vi "LvIRKit_SUB_GetIRKitIPbyName.vi"(8 "error in (no error)":errorcluster caption="エラー入力（エラーなし）", 11 "IRKit name":string="IRKitA741") -> (0 "error out":errorcluster caption="エラー出力", 1 "IP":string)   [LabVIEW 2014]
uses:
  <vilib>/regexp/Match Regular Expression.xnode
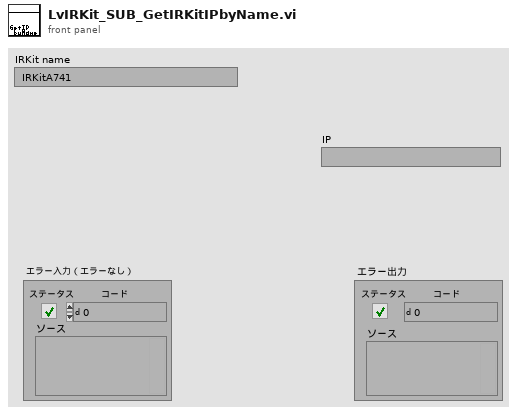
[diagram p1: front panel]
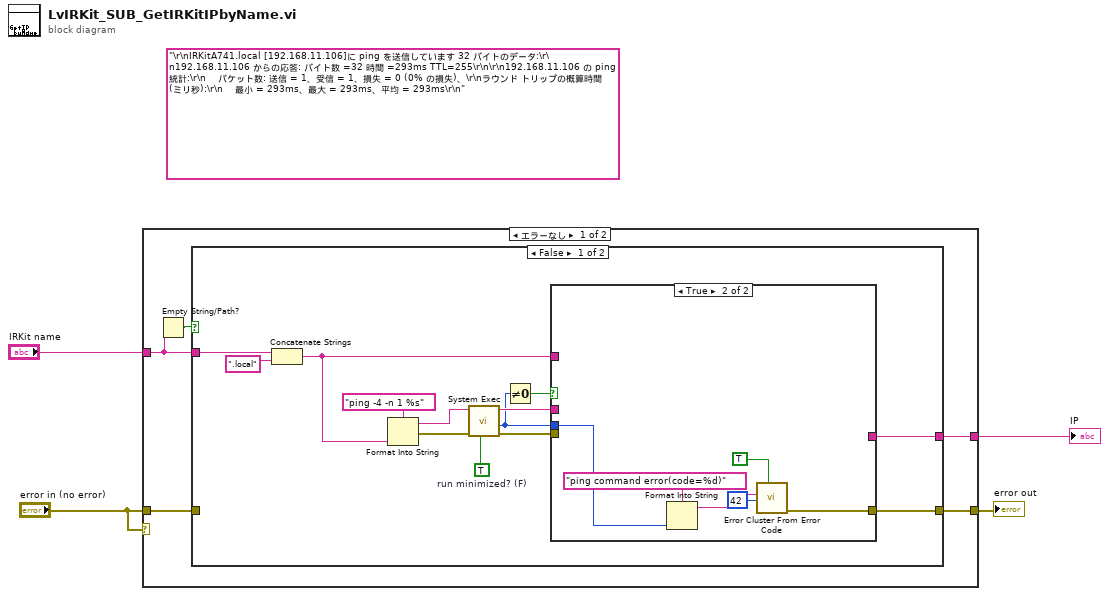
[diagram p0: block diagram]
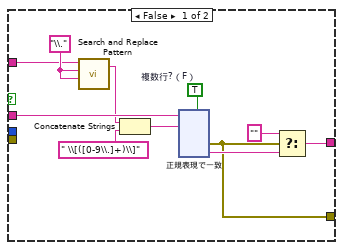
[diagram p2: hidden frame]
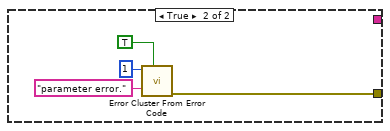
[diagram p3: hidden frame]
diagram:
  (unwired) "\r\nIRKitA741.local [192.168.11.106]に ping を送信しています 32 バイトのデータ:\r\n192.168.11.106 からの応答: バイト数 =32 時間 =293ms TTL=255\r\n\r\n192.168.11.106 の ping 統計:\r\n    パケット数: 送信 = 1、受信 = 1、損失 = 0 (0% の損失)、\r\nラウンド トリップの概算時間 (ミリ秒):\r\n    最小 = 293ms、最大 = 293ms、平均 = 293ms\r\n"
  n1 = case shown="エラーなし" "error in (no error)" {
    tunnel: "IRKit name" -> [w8 _]
    tunnel: [w9 _] -> w3
    tunnel: "error in (no error)" -> [w6 w160]
    tunnel: [w5 w160] -> w1
    frame No Error {
      n2 = Empty String/Path?(string/path=w8) -> (empty?=w7:bool)
      n3 = case shown="FALSE" w7 {
        tunnel: w8 -> [w18 _]
        tunnel: [w15 _] -> w9
        tunnel: w6 -> [_ _]
        tunnel: [w12 w157] -> w5
        frame False {
          w14 = TRUE  # run minimized? (F)
          n4 = Concatenate Strings(w18, ".local" ("IRKit name")) -> (w16:string)
          n5 = Format Into String(format string="ping -4 -n 1 %s" ("command line"), w16) -> (resulting string=w20:string, error out=w19:errorcluster)  [unwired: 2 in]
          n6 = call <vilib>:"System Exec.vi"("run minimized? (F)"=w14, "error in (no error)"=w19, "command line"=w20) -> ("error out"=w11:errorcluster, "return code"=w10:i32, "standard output"=w13:string)  [unwired: 5 in, 1 out]
          n7 = Not Equal To 0?(x=w10) -> (x != 0?=w22:bool)
          n8 = case shown="TRUE" w22 {
            tunnel: w13 -> [w28 _]
            tunnel: w16 -> [w32 _]
            tunnel: [w25 _] -> w15
            tunnel: [w23 w155] -> w12
            tunnel: w11 -> [_ _]
            tunnel: w10 -> [_ w153]
            frame False {
              w31 = TRUE  # 複数行?（F）
              w33 = "\\." ("regular expression (\"\")")
              n9 = call <vilib>:"Search and Replace Pattern.vi"("string"=w32, "regular expression (\"\")"=w33, "replace string (\"\")"=w33) -> ("result string"=w27:string)  [unwired: 2 in, 1 out]
              n10 = Concatenate Strings(w27, " \\[([0-9\\.]+)\\]" ("形式文字列")) -> (w29:string)
              n11 = xnode "正規表現で一致"("入力文字列"=w28, "正規表現"=w29, "複数行?（F）"=w31) -> ("エラー出力"=w23:errorcluster, "部分一致 1"=w26:string)  [unwired: 3 in, 4 out]
              n12 = Select(t="", s=w23, f=w26) -> (s? t:f=w25:string)
            }
            frame True {
              n13 = Format Into String(format string="ping command error(code=%d)" ("error message (\"\")"), w153) -> (resulting string=w151:string)  [unwired: 2 in, 1 out]
              n14 = call <vilib>:"Error Cluster From Error Code.vi"("show call chain? (False)"=TRUE, "error message (\"\")"=w151, "error code (0)"=42) -> ("error out"=w155:errorcluster)  [unwired: 6 in]
            }
          }
        }
        frame True {
          n15 = call <vilib>:"Error Cluster From Error Code.vi"("show call chain? (False)"=TRUE, "error message (\"\")"="parameter error." ("error message (\"\")"), "error code (0)"=1) -> ("error out"=w157:errorcluster)  [unwired: 6 in]
        }
      }
    }
    frame Error {
    }
  }
  "IP" <- w3
  "error out" <- w1
